vi "poly VI A.vi"(11 "Numeric":dbl) -> ()   [LabVIEW 2009]
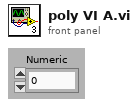
[diagram p1: front panel]
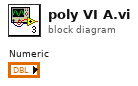
[diagram p0: block diagram]
diagram:
